vi "Custom - Zero.vi"(8 "error in (no error)":errorcluster, 11 "Address":string) -> (0 "error out":errorcluster)   [LabVIEW 2025, in "Interface Functions.lvlib"]
uses:
  Interface Functions.lvlib
  <instrlib>/Agilent U2000 Series/Agilent U2000 Series.lvlib
panel:
  out "read buffer":string
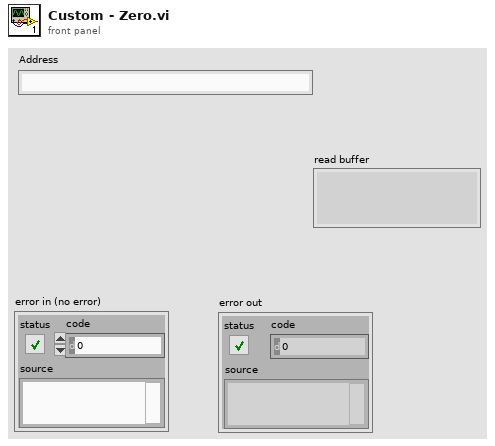
[diagram p1: front panel]
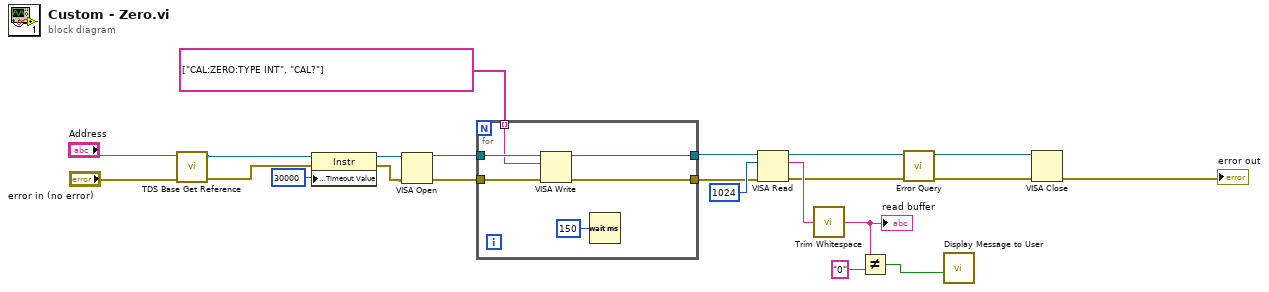
[diagram p0: block diagram]
diagram:
  n1 = call "TDS Base Get Reference.vi"("error in (no error)"="error in (no error)", "Address"="Address") -> ("error out"=w17:errorcluster, "Reference"=w16:refnum<visa-resource-name>)  [unwired: 8 in]
  n2 = property class="Instr"(reference=w16, error in=w17, "General Settings:Timeout Value"=u32 30000) -> (reference out=w19:refnum<visa-resource-name>, error out=w18:errorcluster)
  n3 = VISA Open(error in (no error)=w18, VISA resource name=w19) -> (VISA resource name=w8:refnum<visa-resource-name>, error out=w7:errorcluster)  [unwired: 3 in]
  n4 = for {
    tunnel: string[] ["CAL:ZERO:TYPE INT", "CAL?"] -> [w25] mode=indexing
    tunnel: w8 -> [w28]
    tunnel: [w27] -> w15
    tunnel: w7 -> [w24]
    tunnel: [w23] -> w9
    n5 = VISA Write(VISA resource name=w28, write buffer=w25, error in (no error)=w24) -> (VISA resource name out=w27:refnum<visa-resource-name>, error out=w23:errorcluster)  [unwired: 1 out]
    n6 = Wait (ms)(milliseconds to wait=u32 150) -> ()  [unwired: 1 out]
  }
  n7 = VISA Read(VISA resource name=w15, byte count=u32 1024, error in (no error)=w9) -> (VISA resource name out=w11:refnum<visa-resource-name>, read buffer=w12:string, error out=w10:errorcluster)  [unwired: 1 out]
  n8 = call <vilib>:"Trim Whitespace.vi"("string"=w12) -> ("trimmed string"=w3:string)  [unwired: 1 in]
  "read buffer" <- w3
  n9 = Not Equal?(x=w3, y="0") -> (x != y?=w1:bool)
  n10 = call <instrlib>:"Error Query.vi"("error in (no error)"=w10, "VISA resource name"=w11) -> ("error out"=w5:errorcluster, "VISA resource name out"=w6:refnum<visa-resource-name>)  [unwired: 8 out]
  n11 = call "Display Message to User"("Enable"=w1) -> ()  [unwired: 9 in, 2 out]
  n12 = VISA Close(VISA resource name=w6, error in (no error)=w5) -> (error out=→"error out":errorcluster)
